vi "System Explorer - Add content to System Explorer library.vi"(8 "error in (no error)":errorcluster, 9 "Extra Page Names":string[](array[string]), 10 "Project Root":path, 11 "CD Wizard - Internal Data":T1) -> (0 "error out":errorcluster, 2 "System Explorer Main VI":path, 3 "Load Help File VI":path)   [LabVIEW 2015, in "NIVS_Consolidated_CDW_MetaDataObj.lvclass"]
doc: "Add all virtual folders and VIs to the System Explorer library."
uses:
  NIVS_Consolidated_CDW_MetaDataObj.lvclass
  Internal data.ctl
  CD System Explorer lvlib.ctl
  Add Item - Type.ctl
  CD System Explorer lvlib.vi
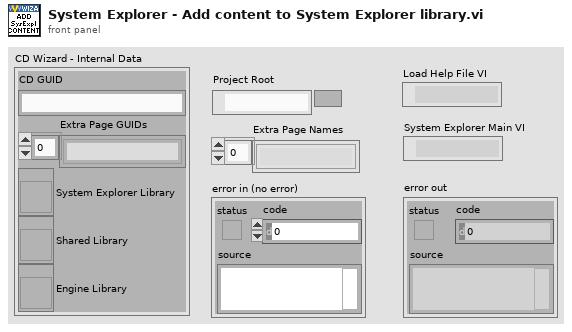
[diagram p1: front panel]
types:
  T1 = typedef "NIVS_Consolidated_CDW_MetaDataObj.lvclass/Internal data.ctl" = cluster{"CD GUID":string, "Extra Page GUIDs":string[], "System Explorer Library":refnum<vi>, "Shared Library":refnum<vi>, "Engine Library":refnum<vi>}
  T2 = typedef "NIVS_Consolidated_CDW_MetaDataObj.lvclass/CD System Explorer lvlib.ctl" = enum16{"LibraryFileName", "LibraryFolderName", "System Explorer.FolderName", "System Explorer.Dynamically Called.FolderName", "System Explorer.Dynamically Called.Extra Pages.FolderName", "System Explorer.Dynamically Called.Extra Pages.TemplatePathAndName", "System Explorer.Dynamically Called.Main Page.VIName", "System Explorer.Dynamically Called.Main Page.TemplatePathAndName", "System Explorer.Dynamically Called.Initialization VI.VIName", "System Explorer.Dynamically Called.Initialization VI.TemplatePathAndName", "System Explorer.SubVI.FolderName", "System Explorer.Types.FolderName", "System Explorer.ActionVIOnCompile.VIName", "System Explorer.ExportConfigRTM.VIName", "System Explorer.LoadHelpFile.VIName"}
  T3 = typedef "NIVS_Consolidated_CDW_MetaDataObj.lvclass/Add Item - Type.ctl" = string
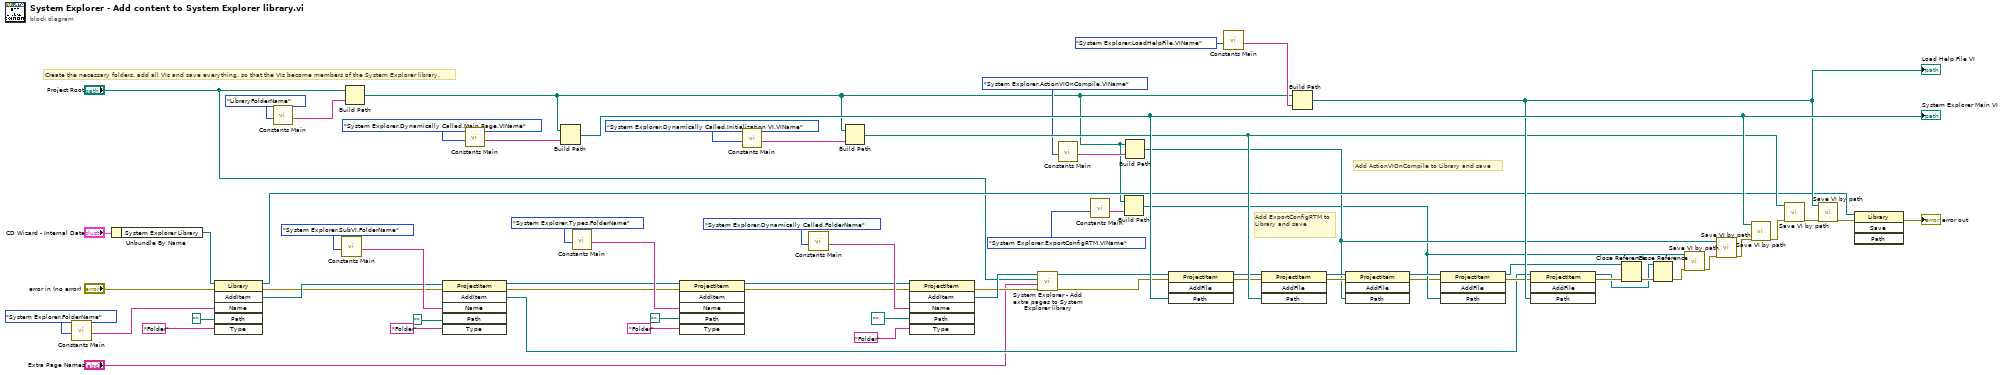
[diagram p0: block diagram]
diagram:
  # "Create the necessary folders, add all VIs and save everything, so that the VIs become members of the System Explorer library."
  # "Add ExportConfigRTM to Library and save"
  # "Add ActionVIOnCompile to Library and save"
  n1 = call-poly "Constants Main.vi"("Action"=CD_System_Explorer_lvlib."System Explorer.FolderName") -> ("Output"=w62:string)  [unwired: 10 in]
  n2 = Unbundle By Name("CD Wizard - Internal Data") -> ("System Explorer Library"=w37:refnum<vi>)
  n3 = invoke class="Library" method="AddItem"(reference=w37, error in="error in (no error)", "Name"=w62, "Path"=path "", "Type"=T3 "Folder" ("Add Item - Type")) -> (reference out=w39:refnum<vi>, error out=w6:errorcluster, "AddItem"=w38:refnum<vi>)  [unwired: 1 in, 3 out]
  n4 = call-poly "Constants Main.vi"("Action"=CD_System_Explorer_lvlib."LibraryFolderName") -> ("Output"=w32:string)  [unwired: 10 in]
  n5 = call-poly "Constants Main.vi"("Action"=CD_System_Explorer_lvlib."System Explorer.SubVI.FolderName") -> ("Output"=w54:string)  [unwired: 10 in]
  n6 = Build Path(base path="Project Root", name or relative path=w32) -> (appended path=w10:path)
  n7 = invoke class="ProjectItem" method="AddItem"(reference=w38, error in=w6, "Name"=w54, "Path"=path "", "Type"=T3 "Folder" ("Add Item - Type")) -> (reference out=w41:refnum<vi>, error out=w5:errorcluster, "AddItem"=w12:refnum<vi>)  [unwired: 1 in, 3 out]
  n8 = call-poly "Constants Main.vi"("Action"=CD_System_Explorer_lvlib."System Explorer.Dynamically Called.Main Page.VIName") -> ("Output"=w60:string)  [unwired: 10 in]
  n9 = Build Path(base path=w10, name or relative path=w60) -> (appended path=w67:path)
  "System Explorer Main VI" <- w67
  n10 = call-poly "Constants Main.vi"("Action"=CD_System_Explorer_lvlib."System Explorer.Types.FolderName") -> ("Output"=w49:string)  [unwired: 10 in]
  n11 = invoke class="ProjectItem" method="AddItem"(reference=w41, error in=w5, "Name"=w49, "Path"=path "", "Type"=T3 "Folder" ("Add Item - Type")) -> (reference out=w40:refnum<vi>, error out=w4:errorcluster)  [unwired: 1 in, 4 out]
  n12 = call-poly "Constants Main.vi"("Action"=CD_System_Explorer_lvlib."System Explorer.Dynamically Called.Initialization VI.VIName") -> ("Output"=w59:string)  [unwired: 10 in]
  n13 = call-poly "Constants Main.vi"("Action"=CD_System_Explorer_lvlib."System Explorer.Dynamically Called.FolderName") -> ("Output"=w44:string)  [unwired: 10 in]
  n14 = Build Path(base path=w10, name or relative path=w59) -> (appended path=w56:path)
  n15 = invoke class="ProjectItem" method="AddItem"(reference=w40, error in=w4, "Name"=w44, "Path"=path "", "Type"=T3 "Folder" ("Add Item - Type")) -> (error out=w34:errorcluster, "AddItem"=w36:refnum<vi>)  [unwired: 1 in, 4 out]
  n16 = call "System Explorer - Add extra pages to System Explorer library.vi"("error in (no error)"=w34, "Extra Page Names"="Extra Page Names", "Project Root"="Project Root", "ProjectItem in"=w36) -> ("error out"=w3:errorcluster, "ProjectItem out"=w35:refnum<vi>)  [unwired: 6 in]
  n17 = call-poly "Constants Main.vi"("Action"=CD_System_Explorer_lvlib."System Explorer.ActionVIOnCompile.VIName") -> ("Output"=w26:string)  [unwired: 10 in]
  n18 = call-poly "Constants Main.vi"("Action"=CD_System_Explorer_lvlib."System Explorer.ExportConfigRTM.VIName") -> ("Output"=w20:string)  [unwired: 10 in]
  n19 = Build Path(base path=w10, name or relative path=w20) -> (appended path=w19:path)
  n20 = Build Path(base path=w10, name or relative path=w26) -> (appended path=w28:path)
  n21 = invoke class="ProjectItem" method="AddFile"(reference=w35, error in=w3, "Path"=w67) -> (reference out=w42:refnum<vi>, error out=w43:errorcluster)  [unwired: 1 in, 2 out]
  n22 = call-poly "Constants Main.vi"("Action"=CD_System_Explorer_lvlib."System Explorer.LoadHelpFile.VIName") -> ("Output"=w11:string)  [unwired: 10 in]
  n23 = invoke class="ProjectItem" method="AddFile"(reference=w42, error in=w43, "Path"=w56) -> (reference out=w31:refnum<vi>, error out=w30:errorcluster)  [unwired: 1 in, 2 out]
  n24 = Build Path(base path=w10, name or relative path=w11) -> (appended path=w66:path)
  "Load Help File VI" <- w66
  n25 = invoke class="ProjectItem" method="AddFile"(reference=w31, error in=w30, "Path"=w28) -> (reference out=w25:refnum<vi>, error out=w16:errorcluster)  [unwired: 1 in, 2 out]
  n26 = invoke class="ProjectItem" method="AddFile"(reference=w25, error in=w16, "Path"=w19) -> (reference out=w15:refnum<vi>, error out=w24:errorcluster)  [unwired: 1 in, 2 out]
  n27 = invoke class="ProjectItem" method="AddFile"(reference=w12, error in=w24, "Path"=w66) -> (reference out=w13:refnum<vi>, error out=w18:errorcluster)  [unwired: 1 in, 2 out]
  n28 = Close Reference(reference=w15, error in (no error)=w18) -> (error out=w22:errorcluster)
  n29 = Close Reference(reference=w13, error in (no error)=w22) -> (error out=w14:errorcluster)
  n30 = call "Save VI by path.vi"("error in (no error)"=w14, "VI path"=w19) -> ("error out"=w23:errorcluster)  [unwired: 9 in]
  n31 = call "Save VI by path.vi"("error in (no error)"=w23, "VI path"=w28) -> ("error out"=w29:errorcluster)  [unwired: 9 in]
  n32 = call "Save VI by path.vi"("error in (no error)"=w29, "VI path"=w67) -> ("error out"=w57:errorcluster)  [unwired: 9 in]
  n33 = call "Save VI by path.vi"("error in (no error)"=w57, "VI path"=w56) -> ("error out"=w9:errorcluster)  [unwired: 9 in]
  n34 = call "Save VI by path.vi"("error in (no error)"=w9, "VI path"=w66) -> ("error out"=w8:errorcluster)  [unwired: 9 in]
  n35 = invoke class="Library" method="Save"(reference=w39, error in=w8) -> (error out=→"error out":errorcluster)  [unwired: 2 in, 3 out]
